vi "UnloadObject.vi"(8 "No Error":errorcluster, 11 "Handle [SDL_SharedObject *]":i64 format="%.0x") -> (0 "Error Out":errorcluster)   [LabVIEW 2024, in "SDL3.lvlib" / "LoadSO.lvlib"]
doc: "<B>Summary</B>\nUnload a shared object from memory.\n\n<B>Remarks</B>\nNote that any pointers from this object looked up through <B>SDL_LoadFunction()</B> will no longer be valid."
uses:
  LoadSO.lvlib
  Lib/SDL3-32.dll
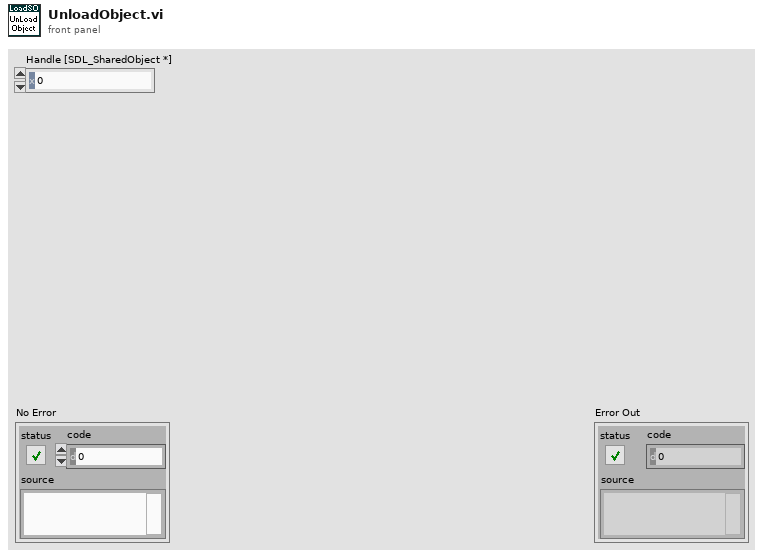
[diagram p1: front panel]
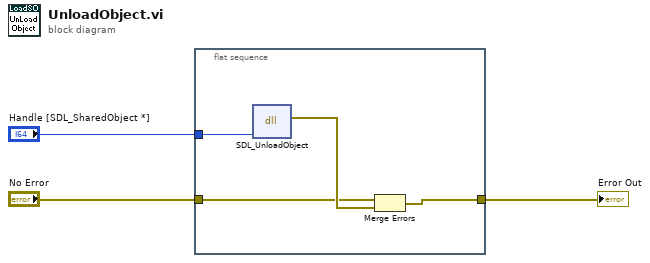
[diagram p0: block diagram]
diagram:
  n1 = flat-sequence {
    tunnel: "Handle [SDL_SharedObject *]" -> [w6]
    tunnel: [w5] -> w2
    tunnel: "No Error" -> [w4]
    frame #0 {
      n2 = dll-call lib="C:/Users/Thomas/Documents/Projects/LV-SDL3/Lib/SDL3-*.*" fn="SDL_UnloadObject"("handle"=w6) -> (error out=w7:errorcluster)  [unwired: 5 in, 1 out]
      n3 = Merge Errors(w4, w7) -> (w5:errorcluster)
    }
  }
  "Error Out" <- w2
